vi "subPopulateExporterSelector.vi"(8 "error in (no error)":errorcluster, 10 "Selection":string, 11 "UIManager in":refnum<class "UIManager.lvclass">) -> (0 "error out":errorcluster, 1 "Display name":string, 2 "Exporter names":string[](array[string]), 3 "UIManager out":refnum<class "UIManager.lvclass">)   [LabVIEW 2020, in "UserInterface.lvlib" / "UIManager.lvclass"]
uses:
  UIManager.lvclass
  UIManager.lvclass/UIManager.ctl
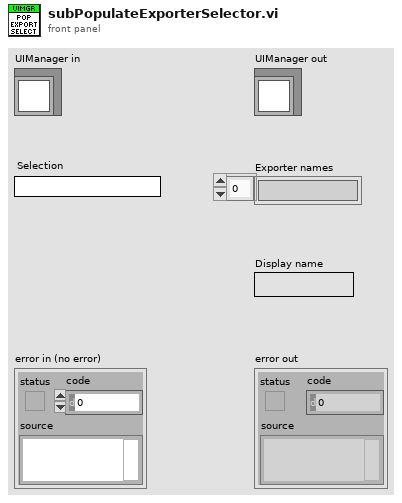
[diagram p1: front panel]
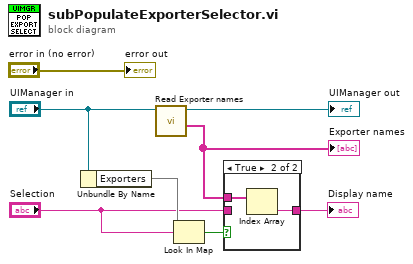
[diagram p0: block diagram]
diagram:
  n1 = Unbundle By Name("UIManager in") -> ("Exporters"=w7:map{string, refnum<class "IExporter.lvclass">})
  n2 = call-dynamic "Read Exporter names.vi"("UIManager in"="UIManager in") -> ("Exporter names"=w1:string[], "UIManager out"=→"UIManager out":refnum<class "UIManager.lvclass">)  [unwired: 9 in]
  "Exporter names" <- w1
  n3 = Look In Map(map=w7, key="Selection") -> (key not found?=w6:bool)  [unwired: 1 in, 1 out]
  n4 = case shown="True" w6 {
    tunnel: w1 -> [_ w11]
    tunnel: [w9 w10] -> w4
    tunnel: "Selection" -> [w9 _]
    frame False {
    }
    frame True {
      n5 = Index Array(array=w11) -> (element=w10:string)  [unwired: 1 in]
    }
  }
  "Display name" <- w4
  "error out" <- "error in (no error)"
